vi "Init HTTP.vi"(8 "error in (no error)":errorcluster, 11 "FormulaLV App in":refnum<class "FormulaG App.lvclass">) -> (0 "error out":errorcluster, 3 "FormulaLV App out":refnum<class "FormulaG App.lvclass">)   [LabVIEW 2020, in "FormulaG.lvlib" / "FormulaG App.lvclass"]
uses:
  FormulaG App.lvclass
  GodotHeaders/GodotHeaders.lvclass
  C:/Program Files (x86)/National Instruments/LabVIEW 2020/vi.lib/IlluminatedG/IG HTTP Server/HTTP Server/Handler/Handler.lvclass
  FormulaG App.lvclass/FormulaG App.ctl
  <vilib>/IlluminatedG/IG HTTP Server/HTTP Server/StandardFileServe/StandardFileServe.lvclass
  <vilib>/IlluminatedG/IG HTTP Server/HTTP Server/Server/Add Connection Handler.vi
  <vilib>/IlluminatedG/IG HTTP Server/HTTP Server/Server/Add Request Handler.vi
  <vilib>/IlluminatedG/IG HTTP Server/HTTP Server/Server/Add Route Handler.vi
  <vilib>/IlluminatedG/IG HTTP Server/HTTP Server/Server/Add Controller Handler.vi
  <vilib>/IlluminatedG/IG HTTP Server/HTTP Server/Server/Add Controller.vi
  <vilib>/IlluminatedG/IG HTTP Server/HTTP Server/Server/Add Response Handler.vi
  <vilib>/IlluminatedG/IG HTTP Server/HTTP Server/Server/Add Complete Handler.vi
  <vilib>/IlluminatedG/IG HTTP Server/HTTP Server/Server/Add Exception Handler.vi
  <vilib>/IlluminatedG/IG HTTP Server/HTTP Server/Connection Handler/Connection Handler.lvclass
  <vilib>/IlluminatedG/IG HTTP Server/HTTP Server/Request Handler/Request Handler.lvclass
  <vilib>/IlluminatedG/IG HTTP Server/HTTP Server/Route Handler/Route Handler.lvclass
  <vilib>/IlluminatedG/IG HTTP Server/HTTP Server/Controller Handler/Controller Handler.lvclass
  <vilib>/IlluminatedG/IG HTTP Server/HTTP Server/Controller/Controller.lvclass
  <vilib>/IlluminatedG/IG HTTP Server/HTTP Server/Response Handler/Response Handler.lvclass
  <vilib>/IlluminatedG/IG HTTP Server/HTTP Server/Complete Handler/Complete Handler.lvclass
  <vilib>/IlluminatedG/IG HTTP Server/HTTP Server/Exception Handler/Exception Handler.lvclass
  <vilib>/IlluminatedG/IG HTTP Server/HTTP Server/Handler/Handler.lvclass
  <vilib>/IlluminatedG/IG HTTP Server/HTTP Server/Server/Server.lvclass
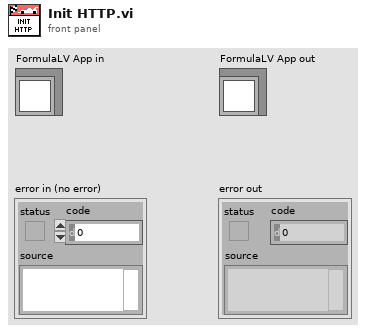
[diagram p1: front panel]
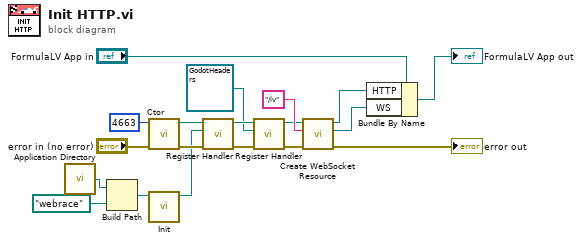
[diagram p0: block diagram]
diagram:
  n1 = call <vilib>:"Application Directory.vi"() -> ("Application Directory"=w17:path)
  n2 = Build Path(base path=w17, name or relative path=path "webrace") -> (appended path=w15:path)
  n3 = call <vilib>:"Ctor.vi"("error in (no error)"="error in (no error)", "HTTP Port (80)"=u16 4663) -> ("error out"=w19:errorcluster, "Server out"=w14:refnum<class "Server.lvclass">)  [unwired: 8 in]
  n4 = call <vilib>:"Init.vi"("Public Root"=w15) -> ("StandardFileServe out"=w13:refnum<class "StandardFileServe.lvclass">)  [unwired: 9 in, 1 out]
  n5 = call <vilib>:"Register Handler.vi"("error in (no error)"=w19, "Handler"=w13, "Server in"=w14) -> ("error out"=w4:errorcluster, "Server out"=w11:refnum<class "Server.lvclass">)  [unwired: 7 in]
  n6 = call <vilib>:"Register Handler.vi"("error in (no error)"=w4, "Handler"=refnum<class "GodotHeaders.lvclass"> refnum ("FormulaLV.lvlib:GodotHeaders.lvclass"), "Server in"=w11) -> ("error out"=w3:errorcluster, "Server out"=w9:refnum<class "Server.lvclass">)  [unwired: 7 in]
  n7 = call <vilib>:"Create WebSocket Resource.vi"("error in (no error)"=w3, "Path"="/lv", "Server in"=w9) -> ("error out"=→"error out":errorcluster, "WS Server"=w1:refnum<class "Websocket Server.lvclass">, "Server out"=w8:refnum<class "Server.lvclass">)  [unwired: 6 in]
  n8 = Bundle By Name(cluster="FormulaLV App in", "HTTP"=w8, "WS"=w1) -> (→"FormulaLV App out":refnum<class "FormulaG App.lvclass">)
